vi "Configure Modulation (IQ).vi"(0 "VISA resource name":refnum<visa-resource-name>, 1 "Enable I/Q Modulator (T:Enable)":bool=TRUE, 2 "Enable Burst Envelop (F:Disable)":bool, 5 "I/Q Source No. (1)":u16(ring)=1 items=["1"=1, "2"=2], 7 "I/Q Source (0: Ext 50 Ohms)":u16(ring) items=["Ext 50 Ohms", "Ext 600 Ohms", "Internal", "Baseband Generator", "Off", "Sum"], 9 "I/Q Signal Source (0: Ext 50 Ohms)":u16(ring) items=["Ext 50 Ohms"=0, "Ext 600 Ohms"=1, "Baseband Generator"=3, "Off"=4], 11 "error in (no error)":errorcluster, 12 "I/Q Phase Polarity (0: Normal)":u16(ring) items=["Normal", "Inverted"], 13 "Summing Ratio (0 dB)":dbl, 14 "Enable High Crest Mode (F:Disable)":bool) -> (4 "VISA resource name out":refnum<visa-resource-name>, 15 "error out":errorcluster)   [LabVIEW 2018, in "Agilent PSG MXG Series.lvlib"]
doc: "Configures the I/Q modulator.\n\n<B>Notes:</B>\n(1) This VI is valid only in E8267C, E8267D, N5162A, N5182A, N5172B, N5182B.\n\n(2) For E8267C, this VI is valid only when the instrument installs <B>Option 002</B> (Internal baseband generator) or <B>Option 602</B> (Digital bus baseband generator)."
uses:
  Agilent PSG MXG Series.lvlib
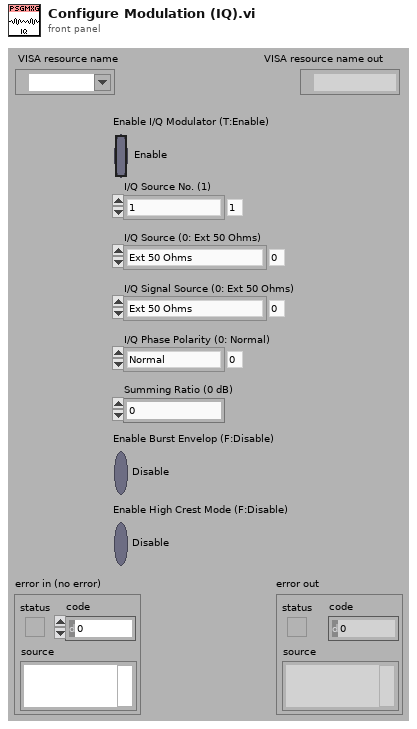
[diagram p1: front panel]
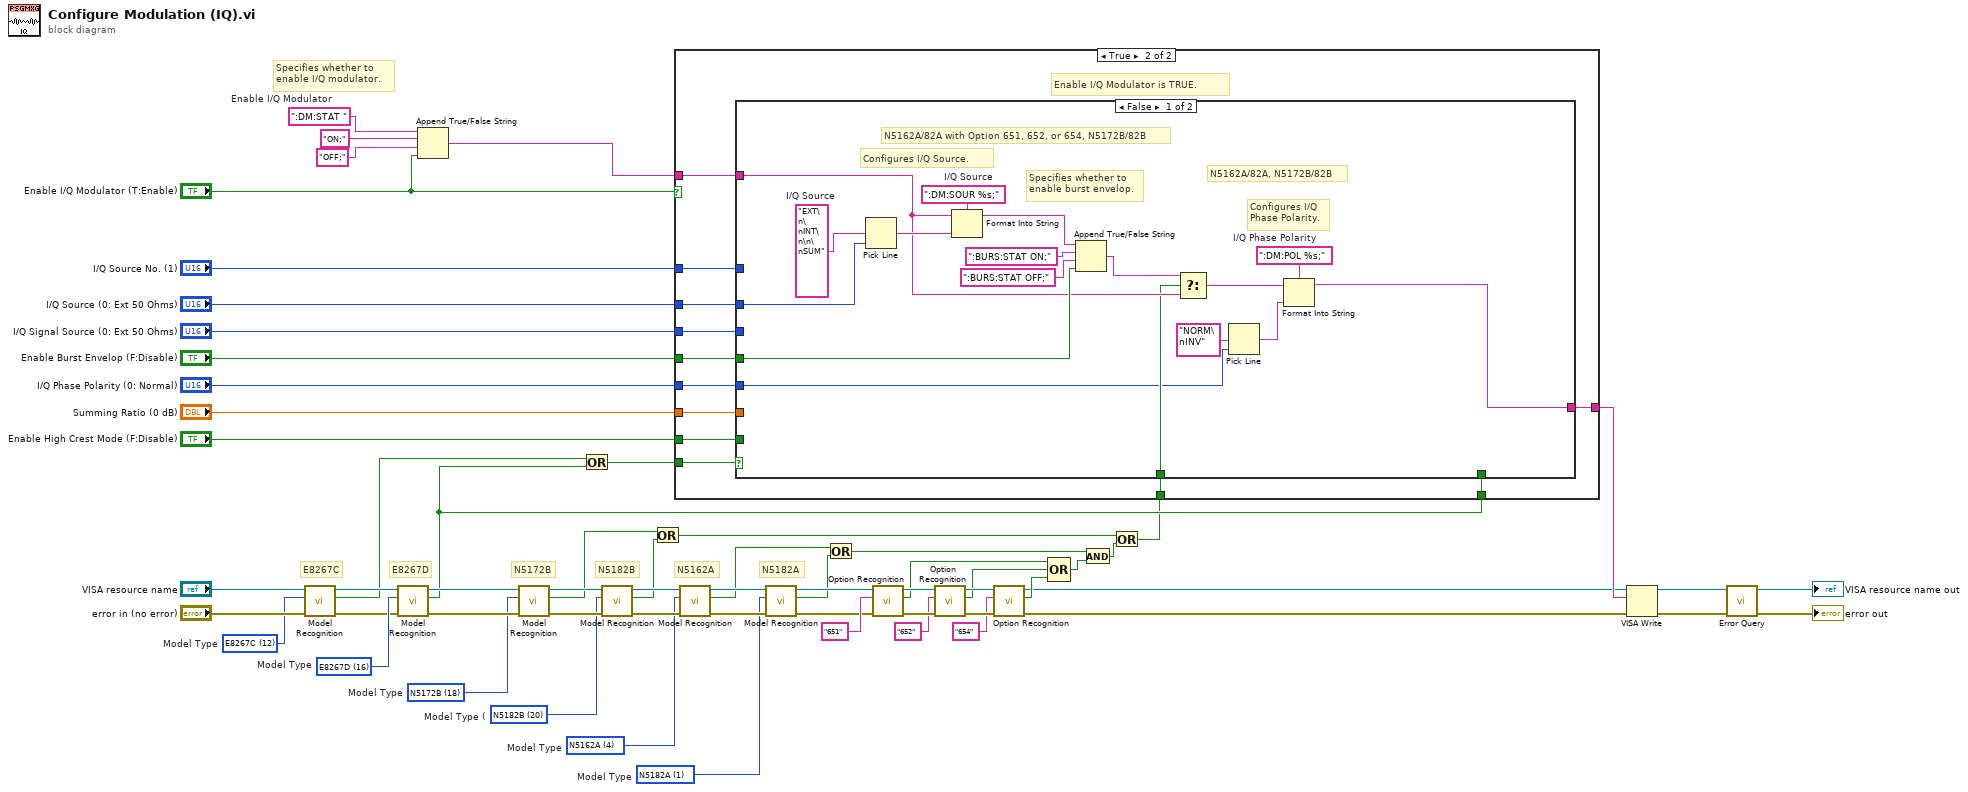
[diagram p0: block diagram]
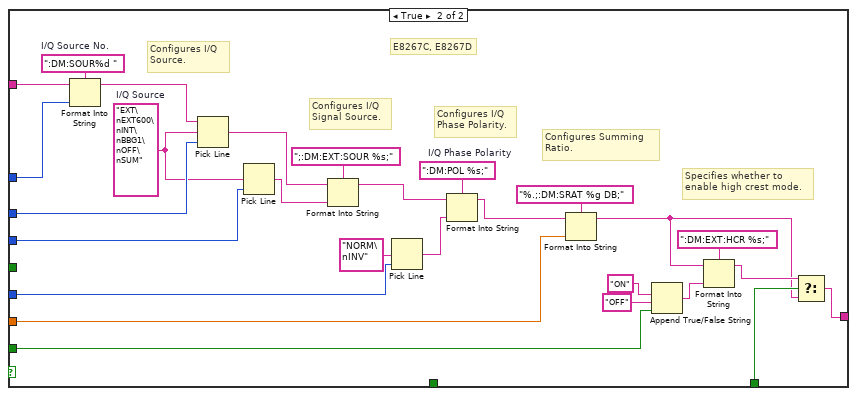
[diagram p3: hidden frame]
diagram:
  w13 = u16 12 items=["N5181A"=0, "N5182A"=1, "N5183A"=2, "N5161A"=3, "N5162A"=4, "E8241A"=5, "E8244A"=6, "E8251A"=7, "E8254A"=8, "E8247C"=10, "E8257C"=11, "E8267C"=12, "E8257D"=15, "E8267D"=16, "N5171B"=17, "N5172B"=18, "N5181B"=19, "N5182B"=20]  # Model Type
  w18 = u16 1 items=["N5181A"=0, "N5182A"=1, "N5183A"=2, "N5161A"=3, "N5162A"=4, "E8241A"=5, "E8244A"=6, "E8251A"=7, "E8254A"=8, "E8247C"=10, "E8257C"=11, "E8267C"=12, "E8257D"=15, "E8267D"=16, "N5171B"=17, "N5172B"=18, "N5181B"=19, "N5182B"=20]  # Model Type
  w19 = u16 4 items=["N5181A"=0, "N5182A"=1, "N5183A"=2, "N5161A"=3, "N5162A"=4, "E8241A"=5, "E8244A"=6, "E8251A"=7, "E8254A"=8, "E8247C"=10, "E8257C"=11, "E8267C"=12, "E8257D"=15, "E8267D"=16, "N5171B"=17, "N5172B"=18, "N5181B"=19, "N5182B"=20]  # Model Type
  w26 = u16 18 items=["N5181A"=0, "N5182A"=1, "N5183A"=2, "N5161A"=3, "N5162A"=4, "E8241A"=5, "E8244A"=6, "E8251A"=7, "E8254A"=8, "E8247C"=10, "E8257C"=11, "E8267C"=12, "E8257D"=15, "E8267D"=16, "N5171B"=17, "N5172B"=18, "N5181B"=19, "N5182B"=20]  # Model Type
  w27 = u16 16 items=["N5181A"=0, "N5182A"=1, "N5183A"=2, "N5161A"=3, "N5162A"=4, "E8241A"=5, "E8244A"=6, "E8251A"=7, "E8254A"=8, "E8247C"=10, "E8257C"=11, "E8267C"=12, "E8257D"=15, "E8267D"=16, "N5171B"=17, "N5172B"=18, "N5181B"=19, "N5182B"=20]  # Model Type
  w28 = u16 20 items=["N5181A"=0, "N5182A"=1, "N5183A"=2, "N5161A"=3, "N5162A"=4, "E8241A"=5, "E8244A"=6, "E8251A"=7, "E8254A"=8, "E8247C"=10, "E8257C"=11, "E8267C"=12, "E8257D"=15, "E8267D"=16, "N5171B"=17, "N5172B"=18, "N5181B"=19, "N5182B"=20]  # Model Type (
  w61 = ":DM:STAT "  # Enable I/Q Modulator
  # "E8267C"
  # "N5182B"
  # "N5172B"
  # "N5162A"
  # "Specifies whether to\nenable I/Q modulator."
  # "E8267D"
  # "N5182A"
  n1 = call "Model Recognition.vi"("error in (no error)"="error in (no error)", "Model Type (0: N5181A)"=w13, "VISA resource name"="VISA resource name") -> ("error out"=w14:errorcluster, "Is Model Correct"=w12:bool, "VISA resource name out"=w16:refnum<visa-resource-name>)  [unwired: 6 out]
  n2 = call "Model Recognition.vi"("error in (no error)"=w14, "Model Type (0: N5181A)"=w27, "VISA resource name"=w16) -> ("error out"=w29:errorcluster, "Is Model Correct"=w11:bool, "VISA resource name out"=w32:refnum<visa-resource-name>)  [unwired: 6 out]
  n3 = Append True/False String(1:"Enable I/Q Modulator (T:Enable)", 2:"OFF;" ("false string"), 3:"ON;" ("true string"), 4:w61) -> (0:w56:string)
  n4 = call "Model Recognition.vi"("error in (no error)"=w29, "Model Type (0: N5181A)"=w26, "VISA resource name"=w32) -> ("error out"=w30:errorcluster, "Is Model Correct"=w4:bool, "VISA resource name out"=w31:refnum<visa-resource-name>)  [unwired: 6 out]
  n5 = Or(x=w12, y=w11) -> (x .or. y?=w10:bool)
  n6 = call "Model Recognition.vi"("error in (no error)"=w30, "Model Type (0: N5181A)"=w28, "VISA resource name"=w31) -> ("error out"=w25:errorcluster, "Is Model Correct"=w5:bool, "VISA resource name out"=w22:refnum<visa-resource-name>)  [unwired: 6 out]
  n7 = Or(x=w4, y=w5) -> (x .or. y?=w1:bool)
  n8 = call "Model Recognition.vi"("error in (no error)"=w25, "Model Type (0: N5181A)"=w19, "VISA resource name"=w22) -> ("error out"=w24:errorcluster, "Is Model Correct"=w8:bool, "VISA resource name out"=w21:refnum<visa-resource-name>)  [unwired: 6 out]
  n9 = call "Model Recognition.vi"("error in (no error)"=w24, "Model Type (0: N5181A)"=w18, "VISA resource name"=w21) -> ("error out"=w23:errorcluster, "Is Model Correct"=w9:bool, "VISA resource name out"=w20:refnum<visa-resource-name>)  [unwired: 6 out]
  n10 = Or(x=w8, y=w9) -> (x .or. y?=w6:bool)
  n11 = call "Option Recognition.vi"("error in (no error)"=w23, "Option (\"\")"="651" ("Option (\"\")"), "VISA resource name"=w20) -> ("error out"=w42:errorcluster, "Is Option Installed"=w37:bool, "VISA resource name out"=w43:refnum<visa-resource-name>)  [unwired: 6 out]
  n12 = call "Option Recognition.vi"("error in (no error)"=w42, "Option (\"\")"="652" ("Option (\"\")"), "VISA resource name"=w43) -> ("error out"=w39:errorcluster, "Is Option Installed"=w36:bool, "VISA resource name out"=w40:refnum<visa-resource-name>)  [unwired: 6 out]
  n13 = call "Option Recognition.vi"("error in (no error)"=w39, "Option (\"\")"="654" ("Option (\"\")"), "VISA resource name"=w40) -> ("error out"=w33:errorcluster, "Is Option Installed"=w35:bool, "VISA resource name out"=w34:refnum<visa-resource-name>)  [unwired: 6 out]
  n14 = Compound Arithmetic op=OR(w37, w36, w35) -> (w7:bool)
  n15 = And(x=w6, y=w7) -> (x .and. y?=w3:bool)
  n16 = Or(x=w1, y=w3) -> (x .or. y?=w2:bool)
  n17 = case shown="True" "Enable I/Q Modulator (T:Enable)" {
    tunnel: "I/Q Source No. (1)" -> [_ w73]
    tunnel: w56 -> [w62 w74]
    tunnel: "I/Q Source (0: Ext 50 Ohms)" -> [_ w72]
    tunnel: "I/Q Signal Source (0: Ext 50 Ohms)" -> [_ w71]
    tunnel: "Enable Burst Envelop (F:Disable)" -> [_ w69]
    tunnel: "I/Q Phase Polarity (0: Normal)" -> [_ w68]
    tunnel: "Summing Ratio (0 dB)" -> [_ w67]
    tunnel: "Enable High Crest Mode (F:Disable)" -> [_ w64]
    tunnel: w11 -> [_ w66]
    tunnel: [w62 w65] -> w47
    tunnel: w2 -> [_ w70]
    tunnel: w10 -> [_ w63]
    frame False {
      # "Enable I/Q Modulator\nis FALSE."
    }
    frame True {
      # "Enable I/Q Modulator is TRUE."
      n18 = case shown="False" w63 {
        tunnel: w74 -> [w82 w118]
        tunnel: w73 -> [_ w117]
        tunnel: w72 -> [w90 w115]
        tunnel: w71 -> [_ w111]
        tunnel: w70 -> [w81 _]
        tunnel: w69 -> [w84 _]
        tunnel: w68 -> [w76 w104]
        tunnel: w67 -> [_ w101]
        tunnel: w66 -> [_ w96]
        tunnel: [w75 w93] -> w65
        tunnel: w64 -> [_ w92]
        frame False {
          w80 = ":DM:POL %s;"  # I/Q Phase Polarity
          w88 = ":DM:SOUR %s;"  # I/Q Source
          w91 = "EXT\n\nINT\n\n\nSUM"  # I/Q Source
          # "N5162A/82A, N5172B/82B"
          # "Configures I/Q\nPhase Polarity."
          # "Specifies whether to\nenable burst envelop."
          # "Configures I/Q Source."
          # "N5162A/82A with Option 651, 652, or 654, N5172B/82B"
          n19 = Pick Line(multi-line string=w91, line index=w90) -> (output string=w89:string)  [unwired: 1 out]
          n20 = Format Into String(format string=w88, initial string=w82, w89) -> (resulting string=w85:string)  [unwired: 1 in, 1 out]
          n21 = Append True/False String(1:w84, 2:":BURS:STAT OFF;" ("true string"), 3:":BURS:STAT ON;" ("true string"), 4:w85) -> (0:w83:string)
          n22 = Select(t=w83, s=w81, f=w82) -> (s? t:f=w79:string)
          n23 = Pick Line(multi-line string="NORM\nINV", line index=w76) -> (output string=w78:string)  [unwired: 1 out]
          n24 = Format Into String(format string=w80, initial string=w79, w78) -> (resulting string=w75:string)  [unwired: 1 in, 1 out]
        }
        frame True {
          w108 = ":DM:POL %s;"  # I/Q Phase Polarity
          w112 = "EXT\nEXT600\nINT\nBBG1\nOFF\nSUM"  # I/Q Source
          w114 = ":DM:SOUR%d "  # I/Q Source No.
          # "Specifies whether to\nenable high crest mode."
          # "Configures Summing\nRatio."
          # "Configures I/Q\nPhase Polarity."
          # "Configures I/Q\nSignal Source."
          # "Configures I/Q\nSource."
          # "E8267C, E8267D"
          n25 = Format Into String(format string=w114, initial string=w118, w117) -> (resulting string=w116:string)  [unwired: 1 in, 1 out]
          n26 = Pick Line(string ("")=w116, multi-line string=w112, line index=w115) -> (output string=w110:string)
          n27 = Pick Line(multi-line string=w112, line index=w111) -> (output string=w109:string)  [unwired: 1 out]
          n28 = Format Into String(format string=";:DM:EXT:SOUR %s;", initial string=w110, w109) -> (resulting string=w105:string)  [unwired: 1 in, 1 out]
          n29 = Pick Line(multi-line string="NORM\nINV", line index=w104) -> (output string=w107:string)  [unwired: 1 out]
          n30 = Format Into String(format string=w108, initial string=w105, w107) -> (resulting string=w102:string)  [unwired: 1 in, 1 out]
          n31 = Format Into String(format string="%.;:DM:SRAT %g DB;", initial string=w102, w101) -> (resulting string=w94:string)  [unwired: 1 in, 1 out]
          n32 = Append True/False String(1:w92, 2:"OFF" ("false string"), 3:"ON" ("true string")) -> (0:w99:string)  [unwired: 1 out]
          n33 = Format Into String(format string=":DM:EXT:HCR %s;", initial string=w94, w99) -> (resulting string=w95:string)  [unwired: 1 in, 1 out]
          n34 = Select(t=w95, s=w96, f=w94) -> (s? t:f=w93:string)
        }
      }
    }
  }
  n35 = VISA Write(VISA resource name=w34, write buffer=w47, error in (no error)=w33) -> (VISA resource name out=w50:refnum<visa-resource-name>, error out=w49:errorcluster)  [unwired: 1 out]
  n36 = call "Error Query.vi"("error in (no error)"=w49, "VISA resource name"=w50) -> ("error out"=→"error out":errorcluster, "VISA resource name out"=→"VISA resource name out":refnum<visa-resource-name>)  [unwired: 8 out]
